vi "CentripetalAccelConstraint_getMaxVelocity.vi"(8 "Velocity":dbl, 9 "Curvature":dbl, 10 "statePose":T2={"TRANSLATION"={"X"=0.0, "Y"=0.0}, "ROTATION"={"VALUE"=0.0, "COS"=1.0, "SIN"=0.0}} {"ROTATION"."SIN" format="%13.4f"; "ROTATION"."COS" format="%13.4f"; "ROTATION"."VALUE" format="%13.4f"; "TRANSLATION"."Y" format="%14.3f"; "TRANSLATION"."X" format="%14.3f"}, 11 "CENTRIPETAL_ACCEL_CONSTRAINT":T1 {"Max Cent Accel" format="%20.4f"}) -> (3 "absMaxVelocity":dbl)   [LabVIEW 2019, in "Trajectory_Library.lvlib"]
doc: "Return the maximum allowed velocity given the provided conditions.\n\nCalculation comments.\n // ac = v^2 / r\n // k (curvature) = 1 / r\n\n // therefore, ac = v^2 * k\n // ac / k = v^2\n // v = std::sqrt(ac / k)\n\n\nParameters:\n - CentripitalAccelConstraint - Constraint data structure\n - statePose - current traj state Pose\n - curvature - current traj curvature\n - maxVelocity - current traj max velocity\n\nReturns\n - maxVelocity - Maximum allowed velocity."
uses:
  Trajectory_Library.lvlib
  TypeDef/TRANSLATION2D.ctl
  TypeDef/ROTATION2D.ctl
  TypeDef/POSE2D.ctl
  TypeDef/TRAJ_CONSTRAINT_CENTRIPETAL_ACCEL.ctl
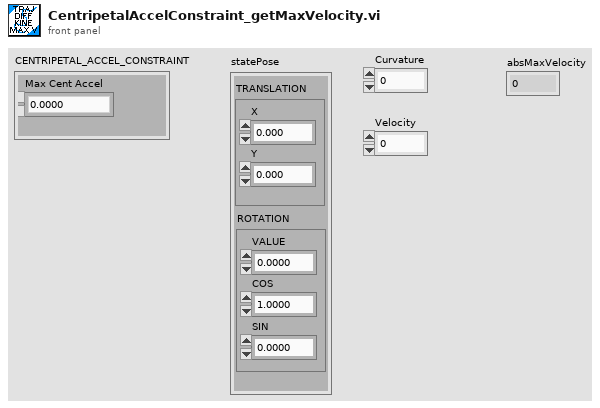
[diagram p1: front panel]
types:
  T1 = typedef "Trajectory_Library.lvlib/TRAJ_CONSTRAINT_CENTRIPETAL_ACCEL.ctl" = cluster{"Max Cent Accel":dbl}
  T2 = typedef "Trajectory_Library.lvlib/POSE2D.ctl" = cluster{"TRANSLATION":T3, "ROTATION":T4}
  T3 = typedef "Trajectory_Library.lvlib/TRANSLATION2D.ctl" = cluster{"X":dbl, "Y":dbl}
  T4 = typedef "Trajectory_Library.lvlib/ROTATION2D.ctl" = cluster{"VALUE":dbl, "COS":dbl, "SIN":dbl}
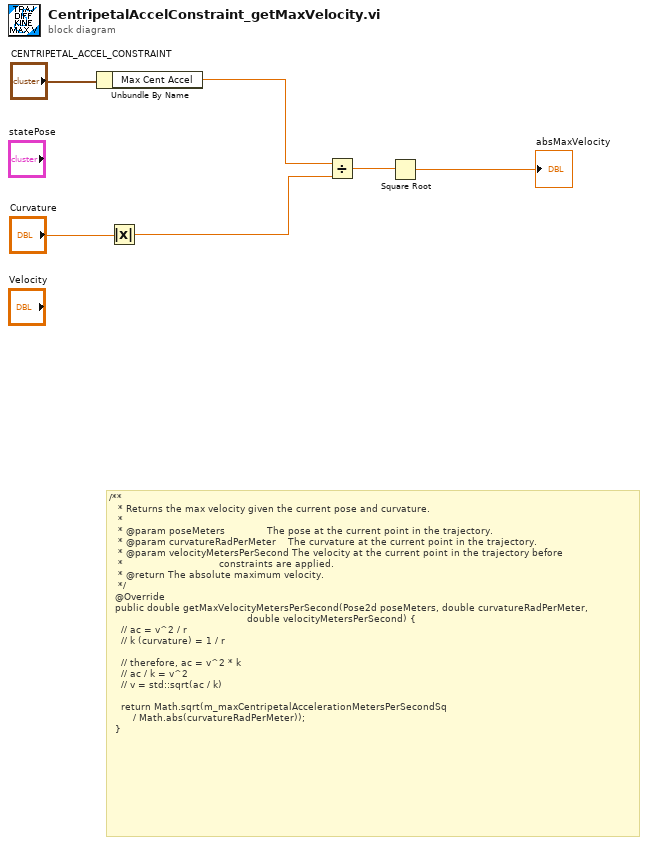
[diagram p0: block diagram]
diagram:
  # "/**\n   * Returns the max velocity given the current pose and curvature.\n   *\n   * @param poseMeters              The pose at the current point in the trajectory.\n   * @param curvatureRadPerMeter    The curvature at the current point in the trajectory.\n   * @param velocityMetersPerSecond The velocity at the current point in the trajectory before\n   *                                constraints are applied.\n   * @return The absolute maximum velocity.\n   */\n  @Override\n  public double getMaxVelocityMetersPerSecond(Pose2d poseMeters, double curvatureRadPerMeter,\n                                              double velocityMetersPerSecond) {\n    // ac = v^2 / r\n    // k (curvature) = 1 / r\n\n    // therefore, ac = v^2 * k\n    // ac / k = v^2\n    // v = std::sqrt(ac / k)\n\n    return Math.sqrt(m_maxCentripetalAccelerationMetersPerSecondSq\n        / Math.abs(curvatureRadPerMeter));\n  }"
  n1 = Unbundle By Name("CENTRIPETAL_ACCEL_CONSTRAINT") -> ("Max Cent Accel"=w4:dbl)
  n2 = Absolute Value(x="Curvature") -> (abs(x)=w3:dbl)
  n3 = Divide(x=w4, y=w3) -> (x/y=w2:dbl)
  n4 = Square Root(x=w2) -> (sqrt(x)=→"absMaxVelocity":dbl)
